vi "S3859061_Task2.vi"() -> ()   [LabVIEW 2020]
panel:
  in  "setting":dbl
  out "alarm":bool
  in  "room C":bool
  in  "room B":bool
  in  "room A":bool
  in  "stop":bool
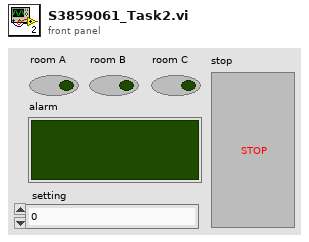
[diagram p1: front panel]
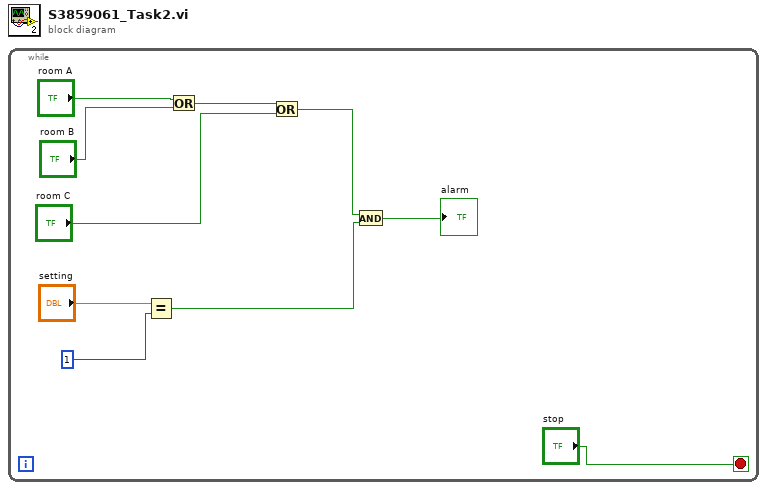
[diagram p0: block diagram]
diagram:
  n1 = while {
    stop <- "stop" stop-if-true
    n2 = Equal?(x="setting", y=1) -> (x = y?=w3:bool)
    n3 = Or(x="room A", y="room B") -> (x .or. y?=w7:bool)
    n4 = Or(x=w7, y="room C") -> (x .or. y?=w2:bool)
    n5 = And(x=w2, y=w3) -> (x .and. y?=→"alarm":bool)
  }
